vi "Configure VSG.vi"(0 "instrument handle in":refnum<k15>, 1 "RFSG port":string, 2 "RFSG Stimulus Mode":T1, 3 "power level (dBm)":dbl=-90.0 format="%.2f", 4 "frequency (Hz)":dbl=100000000.0 format="%.2p", 5 "error in":errorcluster) -> (14 "instrument handle out":refnum<k15>, 19 "error out":errorcluster)   [LabVIEW 2023]
uses:
  <vilib>/niPAEML/Typedefs/RFSG Stimulus Mode.ctl
  <instrlib>/niRFSG/niRFSG.llb/niRFSG Ref Clock Sources.ctl
  <vilib>/niPAEML/PAE Reference.lvclass
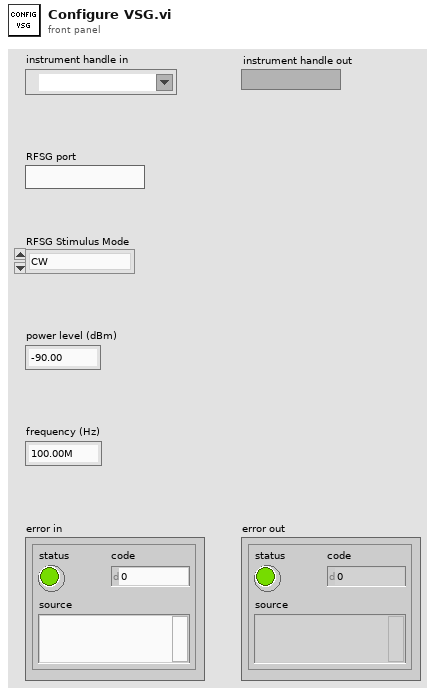
[diagram p1: front panel]
types:
  T1 = typedef "PAE Measurement.lvlib/PAE Reference.lvclass/RFSG Stimulus Mode.ctl" = enum16{"CW", "Pulsed CW"}
  T2 = typedef "niRFSG Ref Clock Sources.ctl" = string
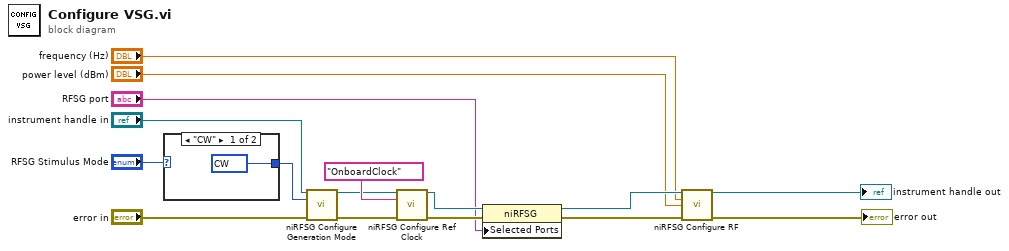
[diagram p0: block diagram]
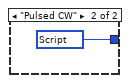
[diagram p2: hidden frame]
diagram:
  n1 = case shown="\"CW\"" "RFSG Stimulus Mode" {
    tunnel: [w17 w18] -> w15
    frame "CW" {
      w17 = 1000 items=["CW"=1000, "Arb Waveform"=1001, "Script"=1002] ("generation mode")
    }
    frame "Pulsed CW" {
      w18 = 1002 items=["CW"=1000, "Arb Waveform"=1001, "Script"=1002] ("generation mode")
    }
  }
  n2 = call <instrlib>:"niRFSG Configure Generation Mode.vi"("instrument handle"="instrument handle in", "generation mode"=w15, "error in"="error in") -> ("instrument handle out"=w13:refnum<k15>, "error out"=w14:errorcluster)  [unwired: 11 out]
  n3 = call <instrlib>:"niRFSG Configure Ref Clock.vi"("instrument handle"=w13, "ref clock source"=T2 "OnboardClock" ("Reference Clock Source"), "error in"=w14) -> ("instrument handle out"=w9:refnum<k15>, "error out"=w8:errorcluster)  [unwired: 1 in, 10 out]
  n4 = property class="niRFSG"(reference=w9, error in=w8, "Selected Ports"="RFSG port") -> (reference out=w7:refnum<k15>, error out=w6:errorcluster)
  n5 = call <instrlib>:"niRFSG Configure RF.vi"("instrument handle"=w7, "frequency (Hz)"="frequency (Hz)", "power level (dBm)"="power level (dBm)", "error in"=w6) -> ("instrument handle out"=→"instrument handle out":refnum<k15>, "error out"=→"error out":errorcluster)  [unwired: 10 in]
